vi "lazoAbierto.vi"() -> ()   [LabVIEW 2011]
panel:
  out "Vo":dbl=0.01048808758431563
  in  "offset":dbl=-0.566
  out "Vo":dynamicdata(graph)=[{"t0"=timestamp(3468875473.047484 s since 1904-01-01), "dt"=1.0, "Y"=[0.01048808758431563]}]
  out "Vo teorico":dbl
  out "RPM":dbl
  in  "Vi":dbl(slide) scale=0.0..5.0
  # "VcEncoder = 12v"
  # "VcMotor = 24v"
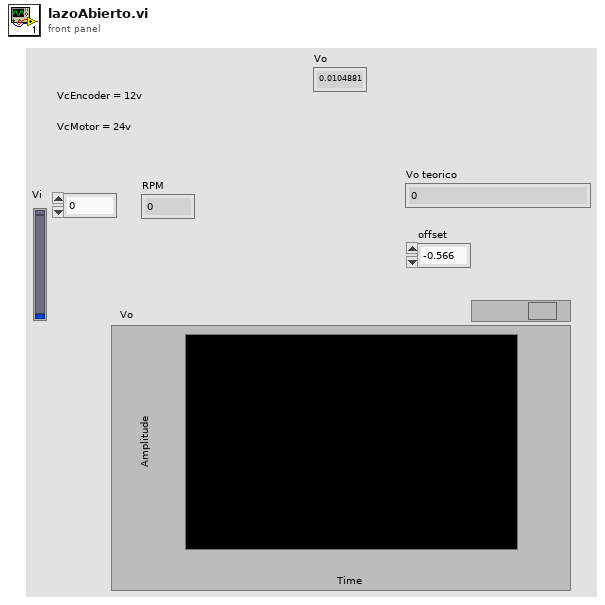
[diagram p1: front panel]
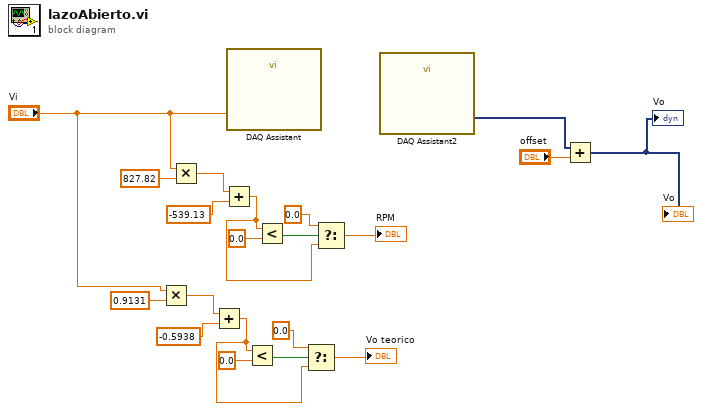
[diagram p0: block diagram]
diagram:
  n1 = Multiply(x="Vi", y=0.9131) -> (x*y=w6:dbl)
  n2 = Multiply(x="Vi", y=827.82) -> (x*y=w19:dbl)
  n3 = Add(x=w6, y=-0.5938) -> (x+y=w12:dbl)
  n4 = Add(x=w19, y=-539.13) -> (x+y=w13:dbl)
  n5 = call "DAQ Assistant"("data"="Vi") -> ()  [unwired: 17 in, 2 out]
  n6 = Less?(x=w12, y=0.0) -> (x < y?=w8:bool)
  n7 = Less?(x=w13, y=0.0) -> (x < y?=w17:bool)
  n8 = Select(t=0.0, s=w8, f=w12) -> (s? t:f=→"Vo teorico":dbl)
  n9 = Select(t=0.0, s=w17, f=w13) -> (s? t:f=→"RPM":dbl)
  n10 = call "DAQ Assistant2"() -> ("data"=w2:dynamicdata)  [unwired: 17 in, 2 out]
  n11 = Add(x=w2, y="offset") -> (x+y=→"Vo" →"Vo":dynamicdata)
